vi "FastPost.vi"(8 "error in (no error)":errorcluster, 10 "Outbound":string, 11 "IPC":i32) -> (0 "error out":errorcluster, 2 "Inbound":string)   [LabVIEW 2013, in "Advanced Plotting Toolkit.lvlib"]
uses:
  Advanced Plotting Toolkit.lvlib
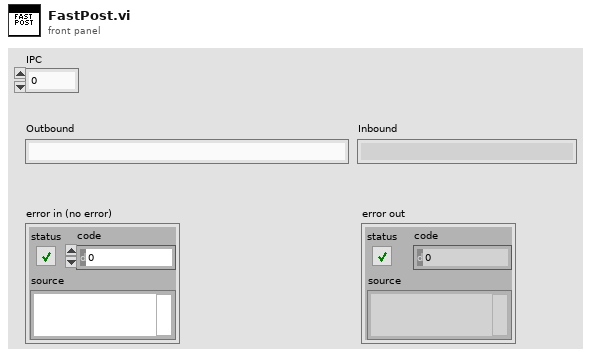
[diagram p1: front panel]
types:
  T1 = enum16{"Standard", "Buffered", "CRLF", "Immediate"}
  T2 = enum16{"big-endian, network order", "native, host order", "little-endian"}
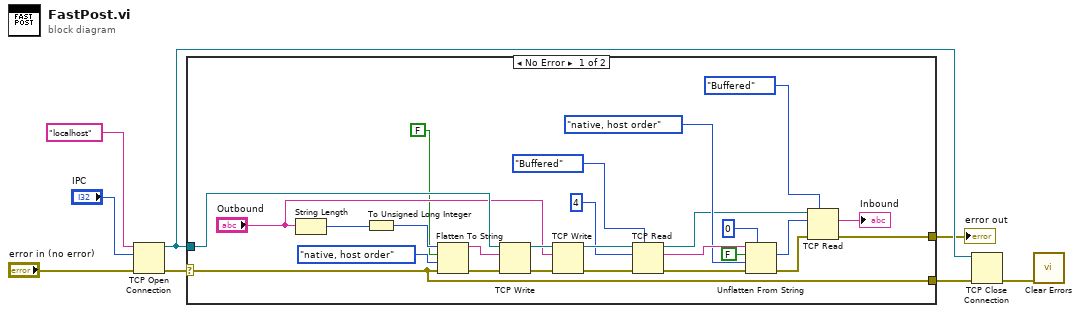
[diagram p0: block diagram]
diagram:
  n1 = TCP Open Connection(address="localhost", remote port or service name="IPC", error in (no error)="error in (no error)") -> (connection ID=w6:refnum<k5>, error out=w7:errorcluster)  [unwired: 2 in]
  n2 = case shown="No Error" w7 {
    selector: w7 -> [w11 w35]
    tunnel: w6 -> [w29 _]
    tunnel: [w12 w35] -> w3
    tunnel: [w11 w35] -> w5
    frame No Error {
      n3 = String Length(string="Outbound") -> (length=w34:i32)
      n4 = To Unsigned Long Integer(number=w34) -> (unsigned 32bit integer=w33:u32)
      n5 = Flatten To String(anything=w33, prepend array or string size? (T)=FALSE, byte order (0:big-endian, network order)=T2."native, host order", error in (no error)=w11) -> (data string=w30:string, error out=w31:errorcluster)  [unwired: 1 out]
      n6 = TCP Write(connection ID=w29, data in=w30, error in (no error)=w31) -> (connection ID out=w27:refnum<k5>, error out=w28:errorcluster)  [unwired: 1 in, 1 out]
      n7 = TCP Write(connection ID=w27, data in="Outbound", error in (no error)=w28) -> (connection ID out=w25:refnum<k5>, error out=w24:errorcluster)  [unwired: 1 in, 1 out]
      n8 = TCP Read(connection ID=w25, bytes to read=4, error in (no error)=w24, 7:T1."Buffered" ("mode (standard)")) -> (connection ID out=w17:refnum<k5>, data out=w21:string, error out=w14:errorcluster)  [unwired: 1 in]
      n9 = Unflatten From String(type=u32 0, binary string=w21, data includes array or string size? (T)=FALSE, byte order (0:big-endian, network order)=T2."native, host order", error in (no error)=w14) -> (value=w16:u32, error out=w13:errorcluster)  [unwired: 1 out]
      n10 = TCP Read(connection ID=w17, bytes to read=w16, error in (no error)=w13, 7:T1."Buffered" ("mode (standard)")) -> (data out=→"Inbound":string, error out=w12:errorcluster)  [unwired: 1 in, 1 out]
    }
    frame Error {
    }
  }
  "error out" <- w3
  n11 = TCP Close Connection(connection ID=w6, error in (no error)=w5) -> (error out=w4:errorcluster)  [unwired: 1 in, 1 out]
  n12 = call <vilib>:"Clear Errors.vi"("error in (no error)"=w4) -> ()  [unwired: 6 in, 1 out]
